vi "Check Firmware.vi"(11 "DCM - RT - RevD in":refnum<class "DCM - RT - RevE.lvclass">) -> (3 "DCM - RT - RevD out":refnum<class "DCM - RT - RevE.lvclass">)   [LabVIEW 2016, in "DCM-Classes.lvlib" / "DCM - RT - RevE.lvclass"]
uses:
  DCM - RT - RevE.lvclass
  D:/PCG/Products/DCM/Software/VeriStand Custom Device/Built/DCM Classes/Pharlap/c/DCM/Rev0/RT/DCM - RT.lvclass
  Rev0/RT/DCM - RT.lvclass/DCM - RT.ctl
  Registers - General.ctl
  Rev0/RT/Write Error.vi
  Rev0/RT/Read FPGA Reference.vi
  <vilib>/rvi/errors/niLvFpgaAdjustHostInterfaceError.vi
  <vilib>/Utility/error.llb/Error Cluster From Error Code.vi
  <vilib>/rvi/interface/nirviMethod/nirviMethod.xnode
  <vilib>/FPGAPlugInAG/Dynamic/niLvFpga_WriteFifo_Dynamic.vi
  <vilib>/rvi/errors/niLvFpgaMergeErrorWithErrorCode.vi
  <vilib>/FPGAPlugInAG/Dynamic/niLvFpga_ReadFifo_Dynamic.vi
  Rev0/RT/DCM - RT.lvclass
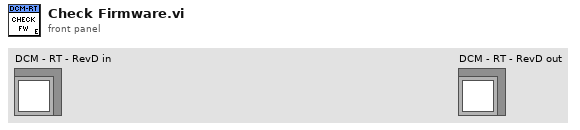
[diagram p1: front panel]
types:
  T1 = typedef "DCM-Classes.lvlib/DCM - RT - RevE.lvclass/Registers - General.ctl" = enum8{"Reserved", "Firmware Major Version", "Firmware Minor Version", "Magic", "Reset", "Control Status 1", "Control Status 2", "Control Status 3", "Control Status 4", "IO Lock Behavior", "Fan Speed 1", "Fan Speed 2", "Fan Speed PW", "FVT Mode", "Control Status FVT", "RS485 Direction", "DI HS Fault Filter Time", "Bleed Fault Filter Time", "Int Filter Time 3", "Int Filter Time 4", "DI HS Fault", "Bleed Fault", "HH Short Fault", "HH Open Fault", "HH Shoot Through Protection", "PFI HS State", "PFI LS State", "PFI Recirc State", "HH-DI Bleed Cmd State", "HH Blank Time", "HH Phase 1 FP", "HH ISeq Dur PS", "Boost DAC Slew", "Reserved 0021", "Reserved 0022", "Reserved 0023", "Reserved 0024", "Reserved 0025", "Reserved 0026", "Reserved 0027", "Reserved 0028", "Reserved 0029", "Reserved 002A", "Reserved 002B", "HH Mode Config Error", "HH Direct Unlock Magic", "HH Direct HS Cmd", "HH Direct LS Cmd", "HH Direct Recirc Cmd", "Boost DAC Primary A1A2", "Boost DAC Primary A3A4", "Boost DAC Primary B3B4", "Boost DAC Primary B1B2", "Boost DAC Secondary A1A2", "Boost DAC Secondary A3A4", "Boost DAC Secondary B3B4", "Boost DAC Secondary B1B2", "Zener PWM Period", "Zener PWM Pulsewidth", "Zener Startup Time"}
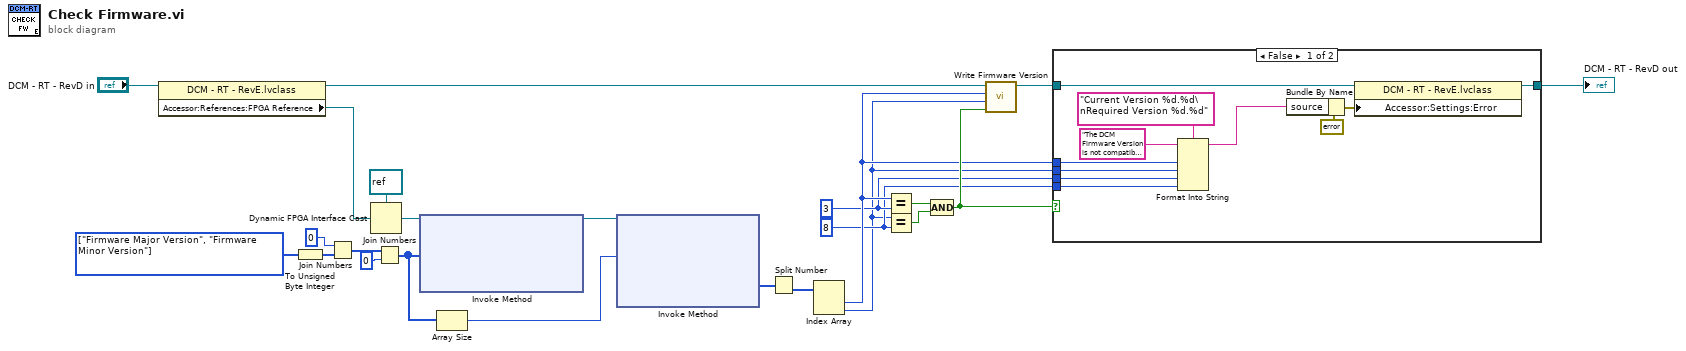
[diagram p0: block diagram]
diagram:
  w2 = u16 8 ("y")
  w3 = u16 3 ("y")
  w16 = T1[] [enum."Firmware Major Version", enum."Firmware Minor Version"] items=["Reserved", "Firmware Major Version", "Firmware Minor Version", "Magic", "Reset", "Control Status 1", "Control Status 2", "Control Status 3", "Control Status 4", "IO Lock Behavior", "Fan Speed 1", "Fan Speed 2", "Fan Speed PW", "FVT Mode", "Control Status FVT", "RS485 Direction", "DI HS Fault Filter Time", "Bleed Fault Filter Time", "Int Filter Time 3", "Int Filter Time 4", "DI HS Fault", "Bleed Fault", "HH Short Fault", "HH Open Fault", "HH Shoot Through Protection", "PFI HS State", "PFI LS State", "PFI Recirc State", "HH-DI Bleed Cmd State", "HH Blank Time", "HH Phase 1 FP", "HH ISeq Dur PS", "Boost DAC Slew", "Reserved 0021", "Reserved 0022", "Reserved 0023", "Reserved 0024", "Reserved 0025", "Reserved 0026", "Reserved 0027", "Reserved 0028", "Reserved 0029", "Reserved 002A", "Reserved 002B", "HH Mode Config Error", "HH Direct Unlock Magic", "HH Direct HS Cmd", "HH Direct LS Cmd", "HH Direct Recirc Cmd", "Boost DAC Primary A1A2", "Boost DAC Primary A3A4", "Boost DAC Primary B3B4", "Boost DAC Primary B1B2", "Boost DAC Secondary A1A2", "Boost DAC Secondary A3A4", "Boost DAC Secondary B3B4", "Boost DAC Secondary B1B2", "Zener PWM Period", "Zener PWM Pulsewidth", "Zener Startup Time"]
  n1 = property class="DCM - RT - RevE.lvclass"(reference="DCM - RT - RevD in") -> (reference out=w22:refnum<class "DCM - RT - RevE.lvclass">, "Accessor:References:FPGA Reference"=w24:refnum<k20>)  [unwired: 1 in, 1 out]
  n2 = To Unsigned Byte Integer(number=w16) -> (unsigned 8bit integer=w20:u8[])
  n3 = Join Numbers(hi=u8 0, lo=w20) -> ((hi.lo)=w18:u16[])
  n4 = Dynamic FPGA Interface Cast(Session In=refnum<k20> refnum ("FPGA Reference"), Type=w24) -> (Session Out=w14:refnum<k20>)
  n5 = Join Numbers(hi=w18, lo=u16 0) -> ((hi.lo)=w13:u32[])
  n6 = xnode "Invoke Method"("FPGA VI Reference In"=w14, "Data"=w13) -> ("FPGA VI Reference Out"=w11:refnum<k20>)  [unwired: 2 in, 2 out]
  n7 = Array Size(array=w13) -> (size(s)=w12:i32)
  n8 = xnode "Invoke Method"("FPGA VI Reference In"=w11, "Number of Elements"=w12) -> ("Data"=w10:u32[])  [unwired: 2 in, 3 out]
  n9 = Split Number(x=w10) -> (lo(x)=w9:u16[])  [unwired: 1 out]
  n10 = Index Array(array=w9) -> (element #1=w4:u16, element #2=w1:u16)  [unwired: 2 in]
  n11 = Equal?(x=w4, y=w3) -> (x = y?=w8:bool)
  n12 = Equal?(x=w1, y=w2) -> (x = y?=w7:bool)
  n13 = Compound Arithmetic op=AND(w8, w7) -> (w6:bool)
  n14 = call "Write Firmware Version.vi"("Setup.Firmware Valid"=w6, "Setup.Firmware Minor"=w1, "Setup.Firmware Major"=w4, "DCM - RT in"=w22) -> ("DCM - RT out"=w5:refnum<class "DCM - RT - RevE.lvclass">)  [unwired: 7 in]
  n15 = case shown="False" w6 {
    tunnel: w5 -> [w35 w36]
    tunnel: [w34 w36] -> w21
    tunnel: w4 -> [w28 _]
    tunnel: w3 -> [w27 _]
    tunnel: w1 -> [w26 _]
    tunnel: w2 -> [w25 _]
    frame False {
      n16 = Format Into String(format string="Current Version %d.%d\nRequired Version %d.%d" ("source"), initial string="The DCM Firmware Version is not compatible with the current DCM Driver Software. Please run the Firmware Update Tool to install the correct version of Firmware.\n\n" ("source"), w28, w26, w27, w25) -> (resulting string=w31:string)  [unwired: 1 in, 1 out]
      n17 = Bundle By Name(cluster=errorcluster {"status"=TRUE, "code"=0, "source"=""} ("Error"), "source"=w31) -> (w32:errorcluster)
      n18 = property class="DCM - RT - RevE.lvclass"(reference=w35, "Accessor:Settings:Error"=w32) -> (reference out=w34:refnum<class "DCM - RT - RevE.lvclass">)  [unwired: 1 in, 1 out]
    }
    frame True {
    }
  }
  "DCM - RT - RevD out" <- w21
